vi "PSTR-Dispose of Data.vi"(0 "Expt State (in) in":T1) -> (4 "Expt State (in) out":T1)   [LabVIEW 2020]
uses:
  CFTS Main Panel SubVIs/CFTS-Experiment State.ctl
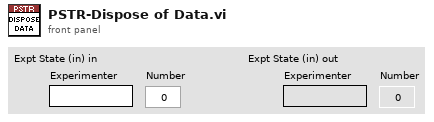
[diagram p1: front panel]
types:
  T1 = typedef "CFTS-Experiment State.ctl" = cluster{"Experimenter":string, "Number":u32, "Right":string, "Left":string, "Data Folder":path, "State File":path, "Version Info":string, "End Exposure Time":dbl, "Exposure Duration":string, "Run #":cluster{"CAP":i16, "ABR":i16, "DP":i16, "VsEP":i16, "MeasSeq":i16, "SubSeq":i16, "SFOAE":i16}}
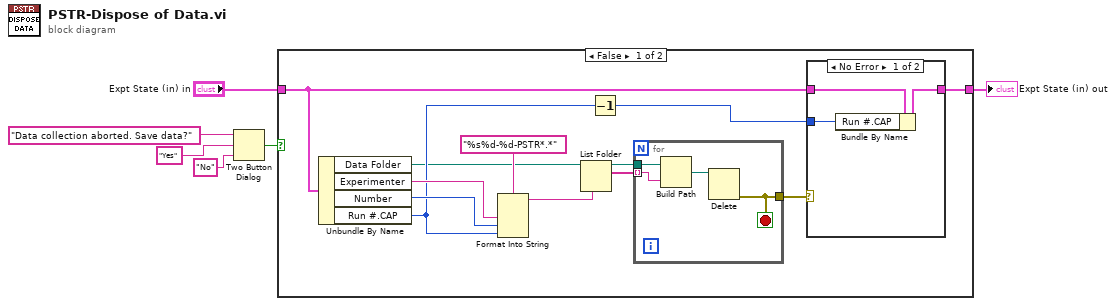
[diagram p0: block diagram]
diagram:
  n1 = Two Button Dialog(message="Data collection aborted. Save data?", 1:"No" ("F button name (\"Cancel\")"), 2:"Yes" ("T button name (\"OK\")")) -> (T button?=w1:bool)
  n2 = case shown="False" w1 {
    tunnel: "Expt State (in) in" -> [w15 w27]
    tunnel: [w14 w27] -> w6
    frame False {
      n3 = Unbundle By Name(w15) -> ("Data Folder"=w11:path, "Experimenter"=w18:string, "Number"=w17:u32, "Run #.CAP"=w12:i16)
      n4 = Format Into String(format string="%s%d-%d-PSTR*.*", w18, w17, w12) -> (resulting string=w10:string)  [unwired: 2 in, 1 out]
      n5 = List Folder(path=w11, pattern=w10) -> (path out=w9:path, filenames=w8:string[])  [unwired: 2 in, 2 out]
      n6 = Decrement(x=w12) -> (x-1=w13:i16)
      n7 = for {
        tunnel: w9 -> [w26]
        tunnel: w8 -> [w25] mode=indexing
        tunnel: [w23] -> w7
        stop <- w23 stop-if-true
        n8 = Build Path(base path=w26, name or relative path=w25) -> (appended path=w24:path)
        n9 = Delete(path (use dialog)=w24) -> (error out=w23:errorcluster)  [unwired: 4 in, 2 out]
      }
      n10 = case shown="No Error" w7 {
        tunnel: w15 -> [w21 w22]
        tunnel: [w20 w22] -> w14
        tunnel: w13 -> [w19 _]
        frame No Error {
          n11 = Bundle By Name(cluster=w21, "Run #.CAP"=w19) -> (w20:T1)
        }
        frame Error {
        }
      }
    }
    frame True {
    }
  }
  "Expt State (in) out" <- w6
